vi "Write Trig Resolution.vi"(8 "error in (no error)":errorcluster, 10 "Trig Resolution":u32, 11 "Configure TRIG Process in":refnum<class "Configure TRIG Process.lvclass">) -> (0 "error out":errorcluster, 3 "Configure TRIG Process out":refnum<class "Configure TRIG Process.lvclass">)   [LabVIEW 2019, in "Trig Process.lvlib" / "Configure TRIG Process.lvclass"]
uses:
  Configure TRIG Process.lvclass
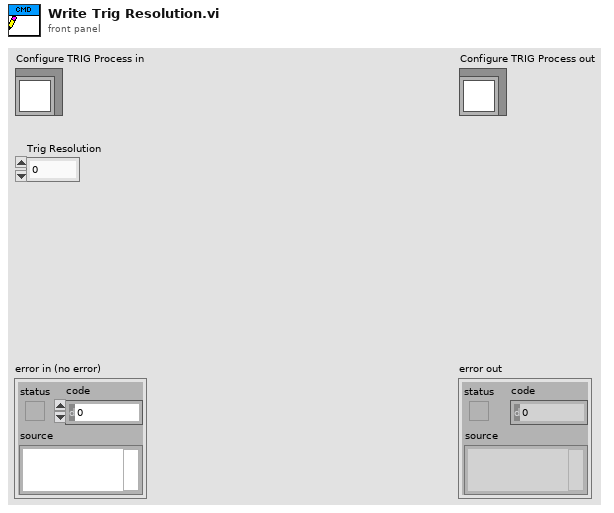
[diagram p1: front panel]
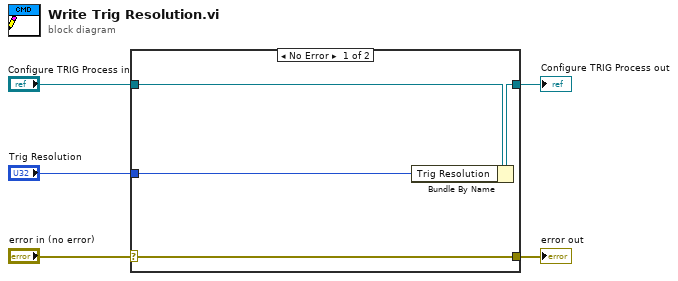
[diagram p0: block diagram]
diagram:
  n1 = case shown="No Error" "error in (no error)" {
    selector: "error in (no error)" -> [w9 w10]
    tunnel: [w9 w10] -> w4
    tunnel: [w7 w11] -> w2
    tunnel: "Configure TRIG Process in" -> [w8 w11]
    tunnel: "Trig Resolution" -> [w6 _]
    frame No Error {
      n2 = Bundle By Name(cluster=w8, "Trig Resolution"=w6) -> (w7:refnum<class "Configure TRIG Process.lvclass">)
    }
    frame Error {
    }
  }
  "error out" <- w4
  "Configure TRIG Process out" <- w2
